vi "Reboot.vi"(8 "error in (no error)":errorcluster, 11 "PF_API in":refnum<class "PF_API.lvclass">) -> (0 "error out":errorcluster, 3 "PF_API out":refnum<class "PF_API.lvclass">)   [LabVIEW 2019, in "PF_API.lvclass"]
uses:
  PF_API.lvclass
  PF_API.lvclass/PF_API.ctl
  <vilib>/httpClient/POSTBuffer.vi
  <vilib>/httpClient/LabVIEWHTTPClient.lvlib
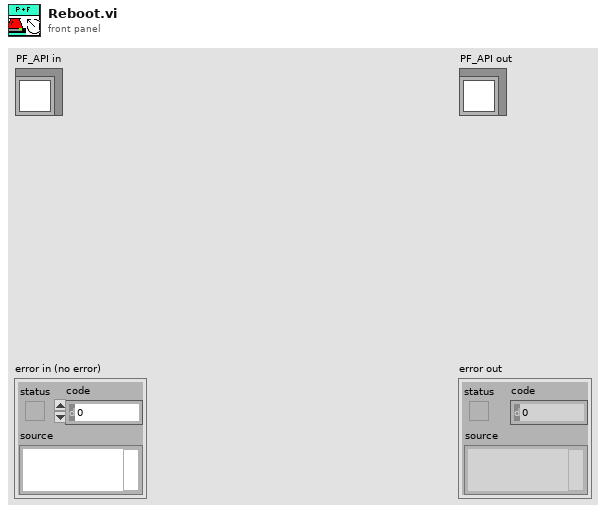
[diagram p1: front panel]
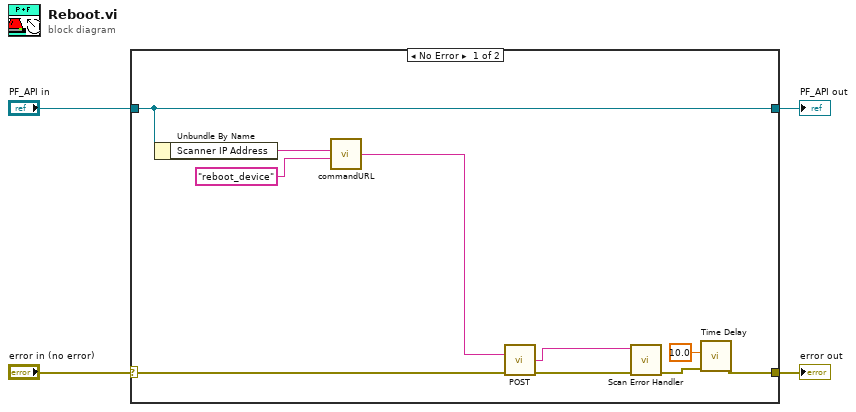
[diagram p0: block diagram]
diagram:
  n1 = case shown="No Error" "error in (no error)" {
    selector: "error in (no error)" -> [w14 w16]
    tunnel: [w9 w16] -> w3
    tunnel: [w13 w15] -> w1
    tunnel: "PF_API in" -> [w13 w15]
    frame No Error {
      n2 = Unbundle By Name(w13) -> ("Scanner IP Address"=w12:string)
      n3 = call "commandURL.vi"("Command String"="reboot_device" ("string"), "Scanner IP Address"=w12) -> ("Command URL"=w6:string)  [unwired: 4 in]
      n4 = call-poly <vilib>:"POST.vi"("url"=w6, "error in (no error)"=w14) -> ("body"=w5:string, "error out"=w7:errorcluster)  [unwired: 10 in, 2 out]
      n5 = call "Scan Error Handler.vi"("Error In"=w7, "HTTP Response"=w5) -> ("Error Out"=w10:errorcluster)  [unwired: 9 in]
      n6 = call "Time Delay"("error in (no error)"=w10, "Delay Time (s)"=10.0) -> ("error out"=w9:errorcluster)  [unwired: 9 in]
    }
    frame Error {
    }
  }
  "error out" <- w3
  "PF_API out" <- w1
